vi "while_v0_v21.vi"() -> ()   [LabVIEW 2009]
panel:
  out "Waveform Chart":dbl(graph)
  in  "Delay (ms)":dbl(slide)=139.04761904761904 scale=0.0..300.0
  out "Secventa":i64=5
  in  "stop":bool
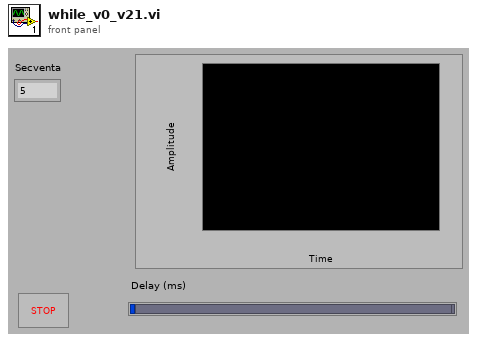
[diagram p1: front panel]
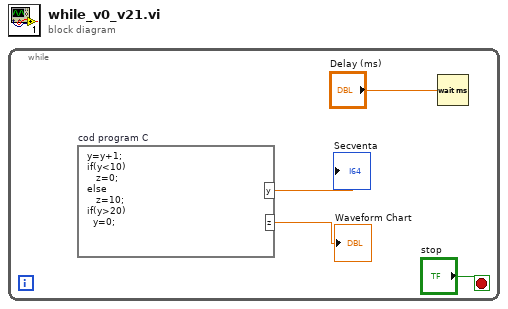
[diagram p0: block diagram]
diagram:
  n1 = while {
    stop <- "stop" stop-if-true
    n2 = formula code="y=y+1;\nif(y<10)\n   z=0;\nelse\n   z=10;\nif(y>20)\n  y=0;" "cod program C"() -> ("y"=→"Secventa":dbl, "z"=→"Waveform Chart":dbl)
    n3 = Wait (ms)(milliseconds to wait="Delay (ms)") -> ()  [unwired: 1 out]
  }
